vi "pathplan.vi"() -> ()   [LabVIEW 2016]
panel:
  out "全场定位错误输出":errorcluster caption="错误输出"
  in  "全场定位串口":refnum<visa-resource-name>="ASRL4::INSTR" caption="全场定位模块"
  out "是否跑完规划路径":bool
  in  "speed_max":dbl=15000.0
  out "路径规划数据写入缓冲区":string
  in  "发送写入":refnum<visa-resource-name>
  in  "车宽的一半":dbl=200.0
  in  "err":dbl[](array[numeric])
  out "起点监视":sgl[](array[numeric])
  out "全场定位缓冲区监视器":string
  in  "目标位置":dbl[](array[numeric])
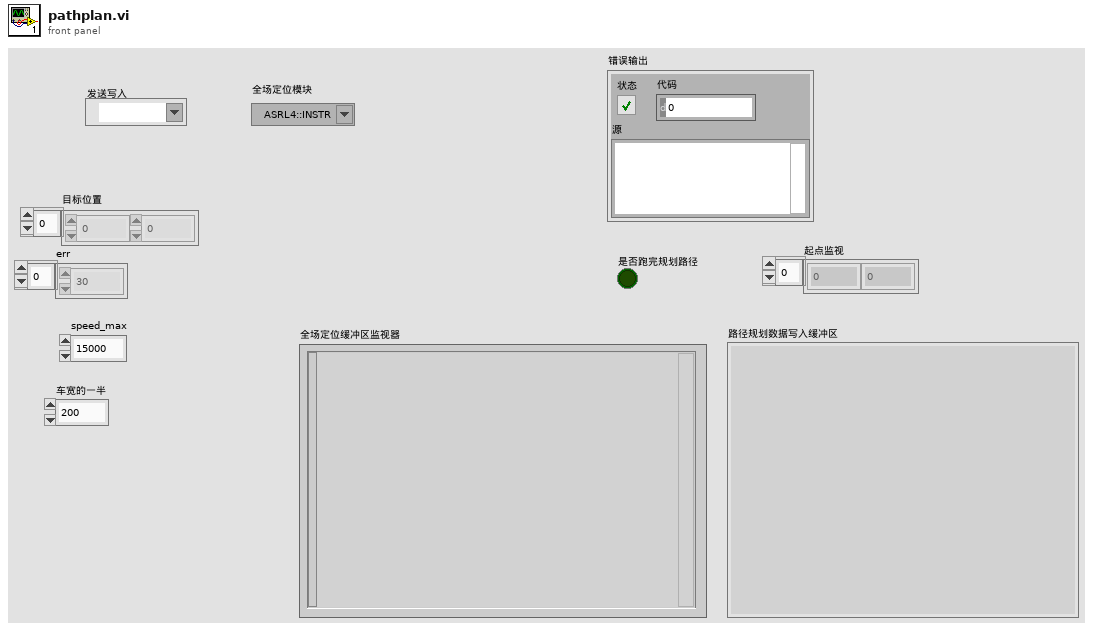
[diagram p1: front panel]
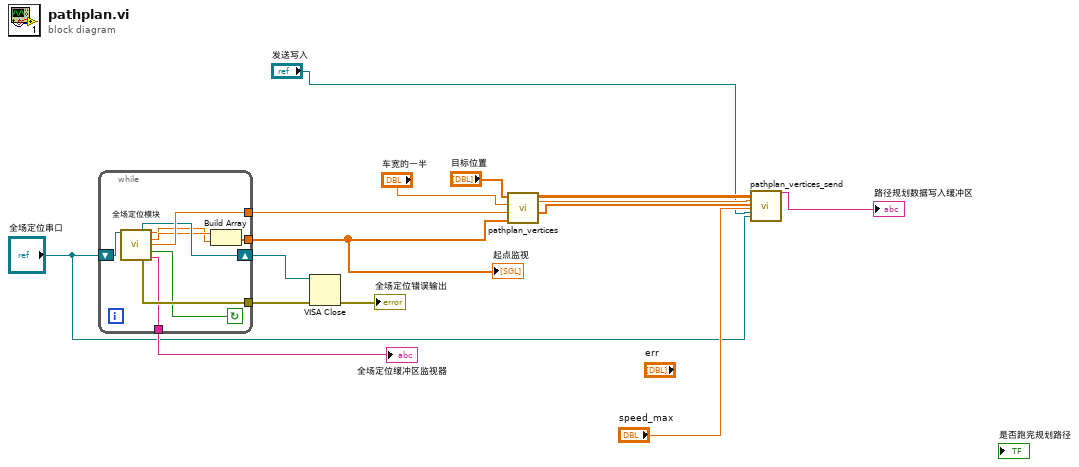
[diagram p0: block diagram]
diagram:
  n1 = while {
    tunnel: [w24] -> w14
    tunnel: [w22] -> w11
    tunnel: [w21] -> w10
    tunnel: [w20] -> w9
    shift-right: [w19] -> w8
    shift-left: "全场定位串口" -> [w23]
    stop <- w18 continue-if-true
    n2 = call "全场定位模块.vi"("VISA resource name"=w23) -> ("VISA资源名称输出"=w19:refnum<visa-resource-name>, "y"=w16:sgl, "x"=w17:sgl, "Zangle"=w20:sgl, "pd"=w18:bool, "错误输出2"=w22:errorcluster, "缓冲区监视器"=w21:string)  [unwired: 8 in]
    n3 = Build Array(w17, w16) -> (w24:sgl[])
  }
  "全场定位缓冲区监视器" <- w10
  "起点监视" <- w14
  n4 = VISA Close(VISA resource name=w8, error in (no error)=w11) -> (error out=→"全场定位错误输出":errorcluster)
  n5 = call "pathplan_vertices.vi"("终点"="目标位置", "车宽的一半"="车宽的一半", "z_angle"=w9, "起点"=w14) -> ("vertices"=w7:dbl[][], "distance_all"=w6:dbl, "angle_all"=w5:dbl[])  [unwired: 3 in, 1 out]
  n6 = call "pathplan_vertices_send.vi"("vertices"=w7, "distance_all"=w6, "angle_all"=w5, "speed_max"="speed_max", "写入串口"="发送写入", "全场定位"="全场定位串口") -> ("路径规划数据写入缓冲区"=→"路径规划数据写入缓冲区":string)  [unwired: 21 in]
